vi "Display_ShowTitleScreen.vi"() -> (16 "SelectedNrOfPlayers":T1)   [LabVIEW 2018]
uses:
  TypDefs/Player_Enum.ctl
  <vilib>/Platform/TimedLoop/XDataNode/timing_clust.ctl
  <vilib>/Platform/TimedLoop/XDataNode/nitl_modes.ctl
  <vilib>/Platform/TimedLoop/XDataNode/wakeup.ctl
  <vilib>/rvi/Emulation/niFpgaSctlEmulationGetInTimedLoop.vi
  <vilib>/rvi/Emulation/niFpgaEmulationReportErrorSimple.vi
  <vilib>/rvi/Emulation/niFpgaGetClockAttributes.vi
  <vilib>/rvi/Emulation/niFpgaCriticalErrorInLSC.vi
  <vilib>/Platform/TimedLoop/XDataNode/XDataNode.xnode
  <vilib>/Platform/TimedLoop/XDataNode/XDNodeRunTimeDep.lvlib
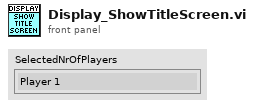
[diagram p1: front panel]
types:
  T1 = typedef "Player_Enum.ctl" = enum16{"Player 1", "Player 2"}
  T2 = typedef "XDNodeRunTimeDep.lvlib/timing_clust.ctl" = cluster{"Expected End [f-1]":u64, "Actual End [f-1]":u64, "Finished Late? [f-1]":bool, "Expected End [i-1]":u64, "Actual End [i-1]":u64, "Finished Late? [i-1]":bool, "Expected Start [i]":u64, "Actual Start [i]":u64, "Expected Start [f]":u64, "Actual Start [f]":u64, "Source Name":string, "Structure Name":string, "Period":i64, "Deadline":i64, "Offset":i64, "Start":i64, "Priority":i32, "Timeout":i32, "Mode":T3, "Wakeup Reason":T4, "Error":errorcluster, "Source Type":string, "Secondary Source Type":string, "Global End Time":u64, "Global Start Time":u64, "Frame Duration":u64, "Iteration Duration":u64, "Assigned CPU":i32, "I/O Scan Engine Mode":u32}
  T3 = typedef "XDNodeRunTimeDep.lvlib/nitl_modes.ctl" = enum32{"No Change", "Process missed periods, maintain original phase", "Discard missed periods, maintain original phase", "Process missed periods, ignore original phase", "Discard missed periods, ignore original phase"}
  T4 = typedef "XDNodeRunTimeDep.lvlib/wakeup.ctl" = enum32{"Normal", "Aborted", "Asynchronous wakeup", "Timing source error", "Timed loop error", "Timeout"}
  T5 = typedef "ActivePixel_Cluster.ctl" = cluster{"h_pixel":i16, "v_pixel":i16}
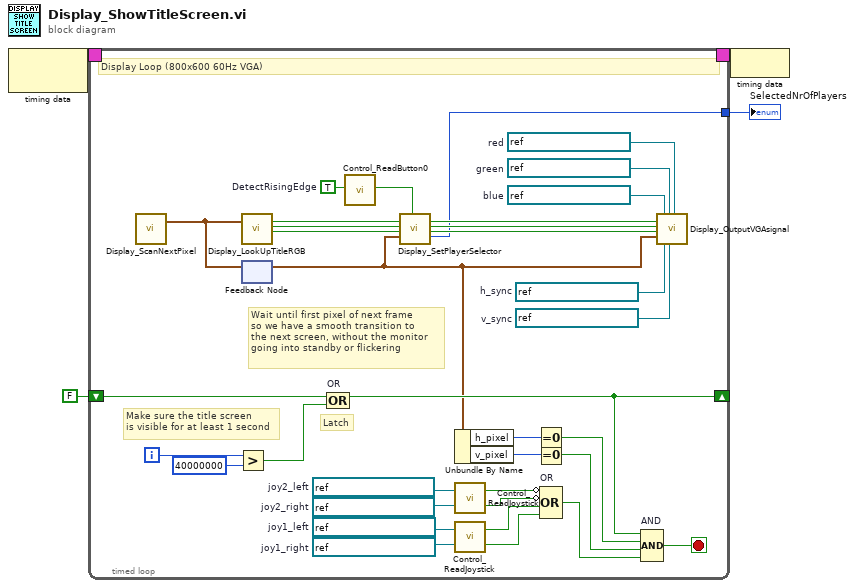
[diagram p0: block diagram]
diagram:
  n1 = node-c288() -> (w4:T2)  [unwired: 1 in]
  n2 = timed-loop {
    timing: w4 -> [_]
    timing-out: [_] -> w3
    tunnel: [w27] -> w2
    shift-right: [w20] -> _
    shift-left: FALSE -> [w22]
    i -> [w24]
    stop <- w25 stop-if-true
    w5 = refnum<k21> "ConnectorC/DIO7"  # joy1_right
    w6 = refnum<k21> "ConnectorC/DIO6"  # joy1_left
    w7 = refnum<k21> "ConnectorB/DIO1"  # joy2_right
    w8 = refnum<k21> "ConnectorB/DIO0"  # joy2_left
    w14 = TRUE  # DetectRisingEdge
    w39 = refnum<k21> "ConnectorC/DIO0"  # red
    w38 = refnum<k21> "ConnectorC/DIO1"  # green
    w37 = refnum<k21> "ConnectorC/DIO2"  # blue
    w36 = refnum<k21> "ConnectorC/DIO4"  # v_sync
    w35 = refnum<k21> "ConnectorC/DIO3"  # h_sync
    # "Wait until first pixel of next frame\nso we have a smooth transition to\nthe next screen, without the monitor\ngoing into standby or flickering"
    # "Latch"
    # "Make sure the title screen\nis visible for at least 1 second"
    # "Display Loop (800x600 60Hz VGA)"
    n3 = call "Display_ScanNextPixel.vi"() -> ("ActivePixel"=w34:T5)  [unwired: 18 in, 1 out]
    n4 = Greater?(x=w24, y=40000000) -> (0:w21:bool)
    n5 = call "Display_LookUpTitleRGB.vi"("ActivePixel"=w34) -> ("Red"=w33:bool, "Green"=w32:bool, "Blue"=w31:bool)  [unwired: 16 in]
    n6 = feedback #1() -> (w19:T5)  [unwired: 1 in]
    n7 = feedback-in #1(w34) -> ()
    n8 = Compound Arithmetic op=OR "OR"(w22, w21) -> (w20:bool)
    n9 = call "Control_ReadButton0.vi"("DetectRisingEdge(F)"=w14) -> ("ButtonPressed"=w26:bool)  [unwired: 18 in]
    n10 = call "Display_SetPlayerSelector.vi"("Red in"=w33, "Green in"=w32, "Blue in"=w31, "ActivePixel"=w19, "Toggle?"=w26) -> ("Red out"=w30:bool, "Green out"=w29:bool, "Blue out"=w28:bool, "SelectedNrOfPlayers"=w27:T1)  [unwired: 11 in]
    n11 = Unbundle By Name(w19) -> ("h_pixel"=w18:i16, "v_pixel"=w17:i16)
    n12 = call "Control_ReadJoystick.vi"("joy_left [FPGA DI]"=w8, "joy_right [FPGA DI]"=w7) -> ("Left"=w13:bool, "Right"=w12:bool)  [unwired: 16 in]
    n13 = call "Control_ReadJoystick.vi"("joy_left [FPGA DI]"=w6, "joy_right [FPGA DI]"=w5) -> ("Left"=w11:bool, "Right"=w10:bool)  [unwired: 16 in]
    n14 = Equal To 0?(x=w18) -> (x = 0?=w16:bool)
    n15 = Equal To 0?(x=w17) -> (x = 0?=w15:bool)
    n16 = Compound Arithmetic op=OR "OR"(invert w13, invert w12, w11, w10) -> (w9:bool)
    n17 = Compound Arithmetic op=AND "AND"(w20, w16, w15, w9) -> (w25:bool)
    n18 = call "Display_OutputVGAsignal.vi"("Red"=w30, "Green"=w29, "Blue"=w28, "ActivePixel"=w19, "Blue [FPGA DO]"=w37, "h_sync [FPGA DO]"=w35, "Green  [FPGA DO]"=w38, "v_sync [FPGA DO]"=w36, "Red  [FPGA DO]"=w39) -> ()  [unwired: 11 in]
  }
  "SelectedNrOfPlayers" <- w2
  n19 = node-c288(w3) -> ()
